vi "Subsystem 1.vi"(10 "Select Transfer Function Type":T1(ring), 11 "system input":dbl) -> (2 "Waveform Chart":waveform(dbl)={"t0"=timestamp(9343.2 s since 1904-01-01), "dt"=1.0, "Y"=[0.2633720690985406]}, 3 "System Output":dbl)   [LabVIEW 2020]
uses:
  <vilib>/Simulation/Implementation/Shared/SIMSCR Execution Mode.ctl
  <vilib>/Simulation/Scripting/Companion Diagram/SimConfigNode/SimParams.ctl
  <vilib>/Simulation/Scripting/Companion Diagram/SimConfigNode/_simSolvers.ctl
  <vilib>/Simulation/Param Hierarchy/Typedefs/SIMPH Param Control Actions.ctl
  <vilib>/Simulation/Implementation/Shared/NILVSim_ParamChanged.vi
  <vilib>/Simulation/Implementation/Shared/NILVSIM_BeginStep.vi
  <vilib>/Simulation/Implementation/Shared/SIM Is Init or Final Stage.vi
  <vilib>/Simulation/DataSources/Implementation/NILVSim Signal Generator.llb/SIM Signal Generator (scalar).vi
  <vilib>/Simulation/ContinuousLinear/Implementation/NILVSim Transfer Function Direct.llb/SIM Transfer Function Direct (MIMO).vi
  <vilib>/Simulation/ContinuousLinear/Implementation/NILVSim Transfer Function.llb/SIM Transfer Function Distributor (SISO).vi
  <vilib>/Simulation/ContinuousLinear/Implementation/NILVSim Transfer Function.llb/SIM Transfer Function Collector (SISO).vi
  <vilib>/Simulation/ContinuousLinear/Implementation/NILVSim Transport Delay.llb/SIM Transport Delay Direct (scalar).vi
  <vilib>/Simulation/ContinuousLinear/Implementation/NILVSim Transfer Function Direct.llb/SIM Transfer Function Direct (SISO).vi
  <vilib>/Simulation/SignalDisplay/Implementation/NILVSim Time Waveform.llb/SIM Time Waveform (scalar).vi
  <vilib>/Simulation/Implementation/Shared/NILVSim_Manager.vi
  <vilib>/Utility/error.llb/Clear Errors.vi
  <vilib>/Simulation/Implementation/Shared/NILVSim_FinalizeModel.vi
  <vilib>/Simulation/Implementation/Shared/SIM Unbundle Sim Info.vi
  <vilib>/Simulation/Implementation/Shared/SIMSH Read Queue.vi
  <vilib>/Simulation/Implementation/Shared/NILVSim_Initialize.vi
  <vilib>/Simulation/Utility/Implementation/NILVSim Get Time and IsAcceptedStep.vi
  <vilib>/Simulation/Implementation/Shared/NILVSim_GetModelError.vi
  <vilib>/Simulation/Implementation/Shared/SIM SimErrorHandler.vi
  <vilib>/Simulation/Implementation/Shared/SIM Bundle Sim Info.vi
  <vilib>/Simulation/Scripting/Companion Diagram/SimConfigNode/SimDog.xnode
  <vilib>/Simulation/Implementation/XNodeFramework/SimXNode/SimX.xnode
  <vilib>/Simulation/ContinuousLinear/Implementation/NILVSim Transfer Function.llb/SIM Transfer Function (SISO).vi
  <vilib>/Simulation/Implementation/Shared/NI_SIM_Implementation.lvlib
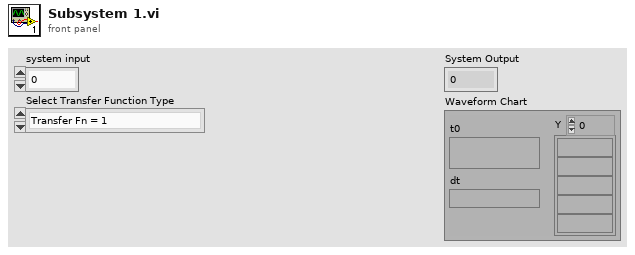
[diagram p1: front panel]
types:
  T1 = enum16{"Transfer Fn = 1", "First Order with Delay", "Second  Order Transfer Fn", "MISO Trf fn example"}
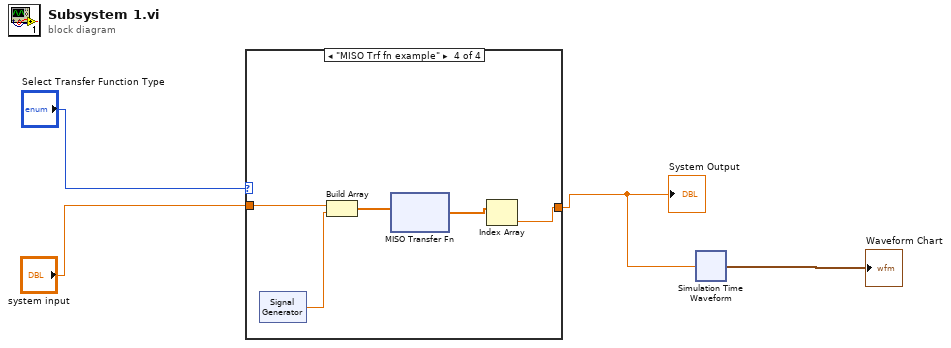
[diagram p0: block diagram]
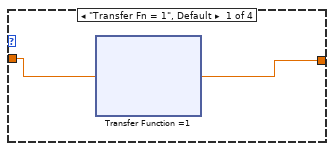
[diagram p2: hidden frame]
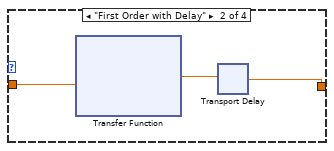
[diagram p3: hidden frame]
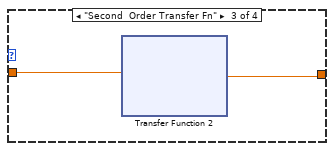
[diagram p4: hidden frame]
diagram:
  n1 = case shown="\"MISO Trf fn example\"" "Select Transfer Function Type" {
    tunnel: "system input" -> [w6 w16 w31 w38]
    tunnel: [w5 w14 w30 w39] -> w1
    frame "Transfer Fn = 1", Default {
      n2 = xnode "Transfer Function =1"("input u(t)"=w6) -> ("output y(t)"=w5:dbl)  [unwired: 4 in, 1 out]
    }
    frame "First Order with Delay" {
      n3 = xnode "Transfer Function"("input u(t)"=w16) -> ("output y(t)"=w15:dbl)  [unwired: 3 in, 1 out]
      n4 = xnode "Transport Delay"("input"=w15) -> ("output"=w14:dbl)  [unwired: 5 in]
    }
    frame "Second  Order Transfer Fn" {
      n5 = xnode "Transfer Function 2"("input u(t)"=w31) -> ("output y(t)"=w30:dbl)  [unwired: 3 in, 1 out]
    }
    frame "MISO Trf fn example" {
      n6 = xnode "Signal Generator"() -> ("output"=w42:dbl)  [unwired: 7 in]
      n7 = Build Array(w38, w42) -> (w41:dbl[])
      n8 = xnode "MISO Transfer Fn"("input u(t)"=w41) -> ("output y(t)"=w40:dbl[])  [unwired: 4 in, 1 out]
      n9 = Index Array(array=w40) -> (element=w39:dbl)  [unwired: 1 in]
    }
  }
  "System Output" <- w1
  n10 = xnode ("Simulation Time Waveform")("Value"=w1) -> ("Waveform Chart"=→"Waveform Chart":waveform(dbl))  [unwired: 1 in]
